vi "Directories.vi"() -> (1 "generated apis":path, 2 "imports":path, 3 "src":path)   [LabVIEW 2024]
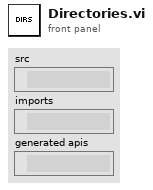
[diagram p1: front panel]
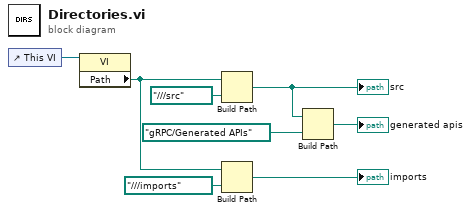
[diagram p0: block diagram]
diagram:
  n1 = control-ref of="This VI"() -> (w8:refnum<vi>)
  n2 = property class="VI"(reference=w8) -> ("Path"=w5:path)  [unwired: 1 in, 2 out]
  n3 = Build Path(base path=w5, name or relative path=path "../../../src") -> (appended path=w3:path)
  "src" <- w3
  n4 = Build Path(base path=w5, name or relative path=path "../../../imports") -> (appended path=→"imports":path)
  n5 = Build Path(base path=w3, name or relative path=path "gRPC/Generated APIs") -> (appended path=→"generated apis":path)
